vi "ReflectArray.vi"(4 "Array In in":i8[][](array[numeric])) -> (1 "Array In out":i8[][](array[numeric]))   [LabVIEW 2020]
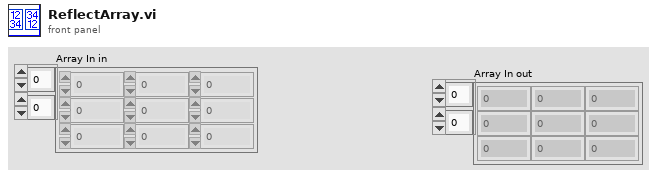
[diagram p1: front panel]
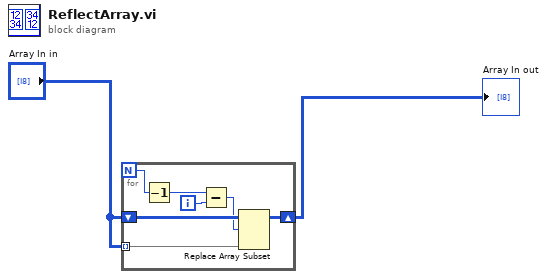
[diagram p0: block diagram]
diagram:
  n1 = for {
    N -> [w4]
    tunnel: "Array In in" -> [w7] mode=indexing
    shift-right: [w8] -> w2
    shift-left: "Array In in" -> [w9]
    i -> [w5]
    n2 = Decrement(x=w4) -> (x-1=w3:i32)
    n3 = Subtract(x=w3, y=w5) -> (x-y=w6:i32)
    n4 = Replace Array Subset(array=w9, new element=w7, index (row)=w6) -> (w8:i8[][])  [unwired: 1 in]
  }
  "Array In out" <- w2
